vi "Reset Index.vi"(8 "error in (no error)":errorcluster, 11 "Action":enum16{"Get", "Set"}(ring)) -> (0 "error out":errorcluster, 3 "Ref Count":u8)   [LabVIEW 2021, in "Utilities.lvlib"]
uses:
  <vilib>/myRIO/Instrument Drivers/Utilities/Utilities.lvlib
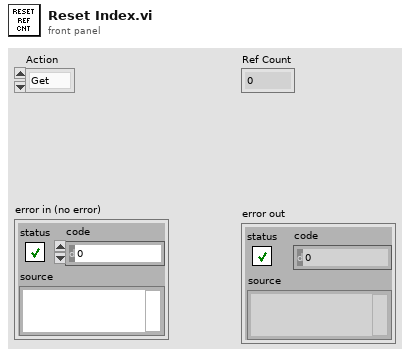
[diagram p1: front panel]
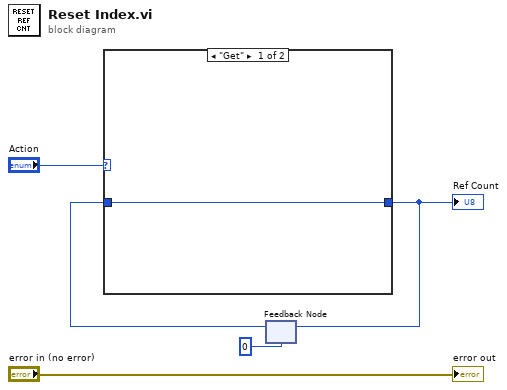
[diagram p0: block diagram]
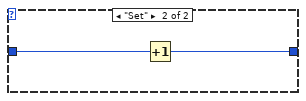
[diagram p2: hidden frame]
diagram:
  n1 = feedback #1(u8 0) -> (w4:u8)
  n2 = case shown="\"Get\"" "Action" {
    tunnel: w4 -> [w6 w8]
    tunnel: [w6 w7] -> w3
    frame "Get" {
    }
    frame "Set" {
      n3 = Increment(x=w8) -> (x+1=w7:u8)
    }
  }
  "Ref Count" <- w3
  n4 = feedback-in #1(w3) -> ()
  "error out" <- "error in (no error)"
